vi "Oscillation_of_MCL_Target-AidanHamiltontestcopy.vi"() -> ()   [LabVIEW 2012]
uses:
  <vilib>/rvi/eio/common/nirviEmuTemplateMethod_errors.vi
  <vilib>/rvi/Emulation/niFpgaSctlEmulationGetInTimedLoop.vi
  <vilib>/rvi/Emulation/niFpgaSctlEmulationGlobalWrite.vi
  <vilib>/eio/EIONode/EIONode.xnode
panel:
  out "Numeric":u64
  in  "Amplitude":i16
  out "Zposition MCL fine":i16
  in  "1/2 the period of oscillation":u32
  in  "Oscillation on/off":bool
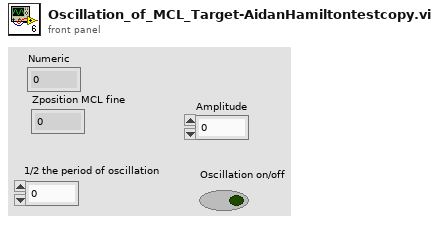
[diagram p1: front panel]
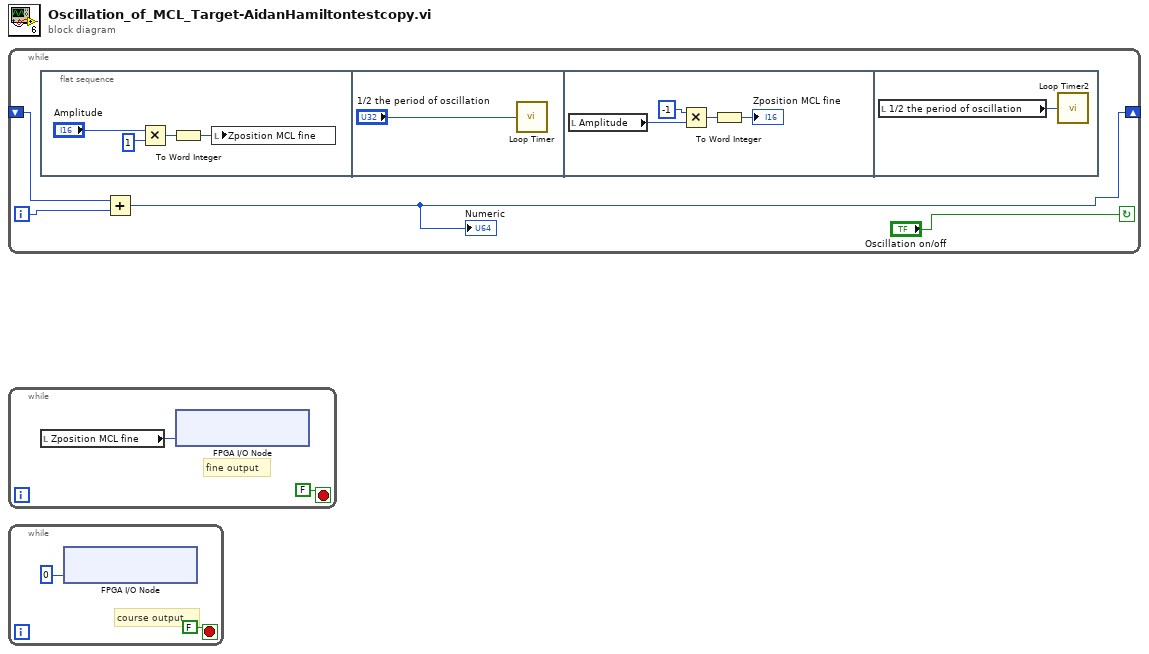
[diagram p0: block diagram]
diagram:
  n1 = while {
    shift-right: [w2] -> _
    shift-left: _ -> [w4]
    i -> [w3]
    stop <- "Oscillation on/off" continue-if-true
    n2 = flat-sequence {
      frame #0 {
        n3 = Multiply(x="Amplitude", y=i16 1) -> (x*y=w6:i16)
        n4 = To Word Integer(number=w6) -> (16bit integer=w5:i16)
        n5 = local write "Zposition MCL fine"(w5) -> ()
      }
      frame #1 {
        n6 = call "Loop Timer"("Count(uSec)"="1/2 the period of oscillation") -> ()  [unwired: 1 out]
      }
      frame #2 {
        n7 = local read "Amplitude"() -> (w13:i16)
        n8 = Multiply(x=i16 -1, y=w13) -> (x*y=w11:i16)
        n9 = To Word Integer(number=w11) -> (16bit integer=→"Zposition MCL fine":i16)
      }
      frame #3 {
        n10 = local read "1/2 the period of oscillation"() -> (w14:u32)
        n11 = call "Loop Timer2"("Count(uSec)"=w14) -> ()  [unwired: 1 out]
      }
    }
    n12 = Add(x=w4, y=w3) -> (x+y=w2:i32)
    "Numeric" <- w2
  }
  n13 = while {
    stop <- FALSE stop-if-true
    # "fine output"
    n14 = local read "Zposition MCL fine"() -> (w16:i16)
    n15 = xnode "FPGA I/O Node"("Connector0/AO7"=w16) -> ()  [unwired: 1 in, 1 out]
  }
  n16 = while {
    stop <- FALSE stop-if-true
    # "course output"
    n17 = xnode "FPGA I/O Node"("Connector0/AO2"=i16 0) -> ()  [unwired: 1 in, 1 out]
  }
